vi "iniciar.vi"() -> ()   [LabVIEW 2016]
uses:
  Control 1.ctl
panel:
  in  "generar":bool
  in  "adquirir":bool
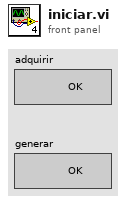
[diagram p1: front panel]
types:
  T1 = typedef "Control 1.ctl" = enum16{"inicio", "espera", "adquirir", "generar", "paro", "reporte1", "reporte2", "reporte3"}
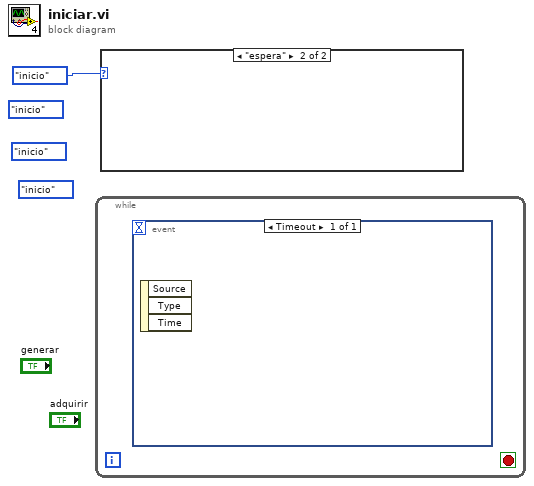
[diagram p0: block diagram]
diagram:
  (unwired) Control_1."inicio" ("Enum")
  (unwired) Control_1."inicio" ("Enum")
  (unwired) Control_1."inicio" ("Enum")
  n1 = while {
    stop <- _ stop-if-true
    n2 = event shown="[0] Timeout" {
      selector: _ -> [_]
      dyn-events: _ -> [_]
      timeout: _ -> [_]
      event Timeout {
        n3 = event-data() -> ()  [unwired: 1 in, 3 out]
      }
    }
  }
  n4 = case shown="\"espera\"" Control_1."inicio" ("Enum") {
    frame "inicio", Default {
    }
    frame "espera" {
    }
  }
